vi "Log Error.vi"(7 "Write to Terminal":bool, 8 "error in (no error)":errorcluster, 11 "CIFCorePlugin in":refnum<class "CIFCorePlugin.lvclass">) -> (0 "error out":errorcluster, 3 "CIFCorePlugin out":refnum<class "CIFCorePlugin.lvclass">)   [LabVIEW 2021, in "CIFCorePlugin.lvclass"]
uses:
  CIFCorePlugin.lvclass
  CIFCorePlugin.lvclass/CIFCorePlugin.ctl
  CIFUtilities/CIFLogs/Typedef/Message Type.ctl
  Accessors/Read Plugin Name.vi
  CIFUtilities/CIFLogs/CIFLogs.lvlib
  CIFCoreCommon/CIFCoreCommon.lvlib
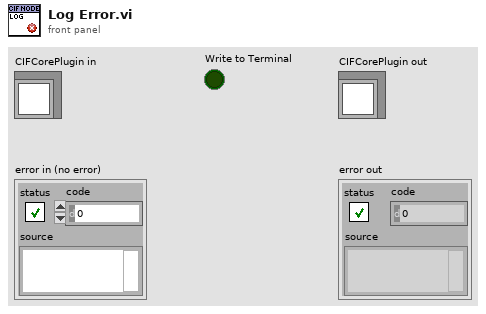
[diagram p1: front panel]
types:
  T1 = typedef "CIFLogs.lvlib/Message Type.ctl" = enum16{"Error", "Information", "Print Terminal", "Configuration"}
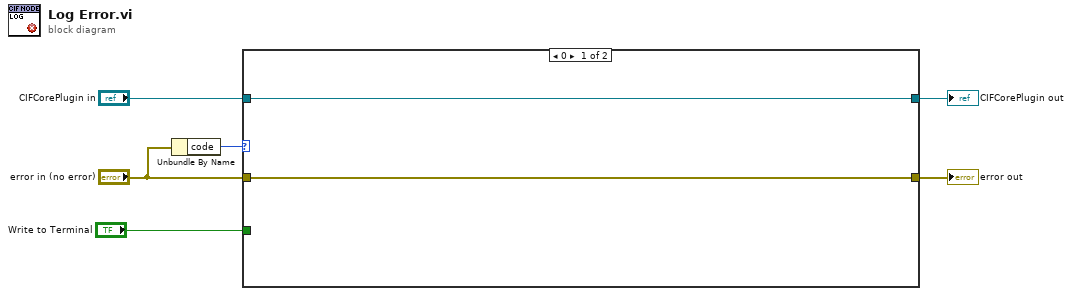
[diagram p0: block diagram]
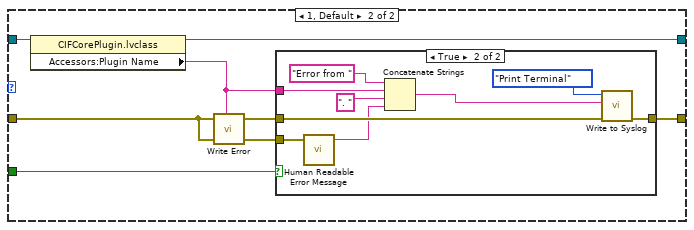
[diagram p2: hidden frame]
diagram:
  n1 = Unbundle By Name("error in (no error)") -> ("code"=w1:i32)
  n2 = case shown="0" w1 {
    tunnel: "CIFCorePlugin in" -> [w8 w15]
    tunnel: [w8 w14] -> w5
    tunnel: [w7 w13] -> w4
    tunnel: "Write to Terminal" -> [_ w11]
    tunnel: "error in (no error)" -> [w7 w10]
    frame 0 {
    }
    frame 1, Default {
      n3 = property class="CIFCorePlugin.lvclass"(reference=w15) -> (reference out=w14:refnum<class "CIFCorePlugin.lvclass">, "Accessors:Plugin Name"=w9:string)  [unwired: 1 in, 1 out]
      n4 = call "Write Error.vi"("error in (no error)"=w10, "Plugin Name"=w9) -> ("cleared error"=w12:errorcluster)  [unwired: 2 in]
      n5 = case shown="True" w11 {
        tunnel: [w16 w25] -> w13
        tunnel: w12 -> [w16 w24]
        tunnel: w10 -> [_ w22]
        tunnel: w9 -> [_ w20]
        frame False {
        }
        frame True {
          n6 = call "Human Readable Error Message.vi"("error in (no error)"=w22) -> ("Human readable error message"=w19:string)  [unwired: 4 in]
          n7 = Concatenate Strings("Error from " ("string"), w20, ". " ("string"), w19) -> (w17:string)
          n8 = call "Write to Syslog.vi"("error in (no error)"=w24, "message"=w17, "CIF Message Type"=Message_Type."Print Terminal") -> ("error out"=w25:errorcluster)  [unwired: 8 in]
        }
      }
    }
  }
  "error out" <- w4
  "CIFCorePlugin out" <- w5
